vi "Create Index Map of Edges.vi"(8 "error in (no error)":errorcluster, 11 "2D Array binary in":refnum<class "2D Array binary.lvclass">) -> (0 "error out":errorcluster, 3 "2D Array binary out":refnum<class "2D Array binary.lvclass">)   [LabVIEW 2024, in "G2CPU Line Profile.lvlib"]
uses:
  G2CPU Line Profile.lvlib
  <vilib>/Natan Biesmans/G2CPU GPU and CPU HPC Toolkit/G2CPU Libraries/Arrays/2DArray/binary/2D Array binary.lvclass
  C:/Program Files/National Instruments/LabVIEW 2025/vi.lib/Natan Biesmans/G2CPU GPU and CPU HPC Toolkit/G2CPU Libraries/Arrays/Array/Array Prototype.lvclass
  C:/Program Files/National Instruments/LabVIEW 2025/vi.lib/Natan Biesmans/G2CPU GPU and CPU HPC Toolkit/G2CPU Libraries/Arrays/2DArray/2D Array Prototype.lvclass
  7be18b7c-d882-49a8-9bf3-9473975a2643.vi
  755dcc6d-d8b2-44ca-8967-bbed7c2483ca.vi
  b529d340-ea47-4164-86f1-e656114a860c.vi
  e5d4ff20-5dd6-4683-aa2a-8e7ba50b1f3d.vi
  d67c9315-a3db-4bd2-ba9f-b6b2c326ac84.vi
  a1422bdd-7d02-45b2-bd73-1aa3fc453463.vi
  be544eb2-5529-4343-82fc-932d6cc08acc.vi
  9e079d64-024a-4165-b95c-f022ae12d1bc.vi
  bbe568f6-b578-42fd-8d12-2a0471a10e1d.vi
  7be18b7c-d882-49a8-9bf3-9473975a2643.vi/e7247370-a01f-465a-ac0e-4dfefcb1bb87.vi
  7be18b7c-d882-49a8-9bf3-9473975a2643.vi/345e91f0-9a5e-4de4-af9c-133346717e4a.vi
  755dcc6d-d8b2-44ca-8967-bbed7c2483ca.vi/08cb2c43-1c8b-4a3a-83bc-b3e8cdef0e3a.vi
  755dcc6d-d8b2-44ca-8967-bbed7c2483ca.vi/f755307d-5806-43cd-9fa2-5ac75ab59def.vi
  755dcc6d-d8b2-44ca-8967-bbed7c2483ca.vi/37397dd5-2c89-4701-b050-64d2f1e61e81.vi
  b529d340-ea47-4164-86f1-e656114a860c.vi/e2b7cdad-9748-47a9-8803-19dad6ab3e2b.vi
  b529d340-ea47-4164-86f1-e656114a860c.vi/edeb7e37-ba5b-4522-b7cc-59d3333e22dd.vi
  e5d4ff20-5dd6-4683-aa2a-8e7ba50b1f3d.vi/f4654d05-beb0-4753-bab7-24376daae318.vi
  e5d4ff20-5dd6-4683-aa2a-8e7ba50b1f3d.vi/a2f9e1c9-c94e-4cd6-9432-cf54c3ac582a.vi
  d67c9315-a3db-4bd2-ba9f-b6b2c326ac84.vi/5fd79b99-6405-4116-b267-99be9ebfbdc8.vi
  d67c9315-a3db-4bd2-ba9f-b6b2c326ac84.vi/f56d75f8-a737-48e1-b5f1-0ddebb8102b6.vi
  d67c9315-a3db-4bd2-ba9f-b6b2c326ac84.vi/f51773da-75cb-4248-9bbd-2a32f0924584.vi
  d67c9315-a3db-4bd2-ba9f-b6b2c326ac84.vi/1de671e1-a703-4849-b735-ab080ea3bfc0.vi
  a1422bdd-7d02-45b2-bd73-1aa3fc453463.vi/f4654d05-beb0-4753-bab7-24376daae318.vi
  a1422bdd-7d02-45b2-bd73-1aa3fc453463.vi/a2f9e1c9-c94e-4cd6-9432-cf54c3ac582a.vi
  9e079d64-024a-4165-b95c-f022ae12d1bc.vi/e9bebd79-1c27-4fc1-b91f-30516104c7f0.vi
  bbe568f6-b578-42fd-8d12-2a0471a10e1d.vi/51c1d4c7-dece-4c02-9cce-b98611dadc4a.vi
  bbe568f6-b578-42fd-8d12-2a0471a10e1d.vi/3d9751b5-328d-444c-aff4-1d084998b389.vi
  b529d340-ea47-4164-86f1-e656114a860c.vi/e2b7cdad-9748-47a9-8803-19dad6ab3e2b.vi/6058dca8-195d-4566-b47b-6d6a1c5af61f.vi
  b529d340-ea47-4164-86f1-e656114a860c.vi/e2b7cdad-9748-47a9-8803-19dad6ab3e2b.vi/6058dca8-195d-4566-b47b-6d6a1c5af61f.vi/77c7badc-ed81-4514-99c1-20d37f4e5ecc.vi
  b529d340-ea47-4164-86f1-e656114a860c.vi/e2b7cdad-9748-47a9-8803-19dad6ab3e2b.vi/6058dca8-195d-4566-b47b-6d6a1c5af61f.vi/eb76fa01-6782-47b4-b34f-9eb474c9cc78.vi
  <vilib>/Natan Biesmans/G2CPU GPU and CPU HPC Toolkit/G2CPU Libraries/Arrays/2DArray/s64/2D Array s64.lvclass
  <vilib>/Natan Biesmans/G2CPU GPU and CPU HPC Toolkit/G2CPU Libraries/Arrays/2DArray/2D Array Prototype.lvclass
  <vilib>/Natan Biesmans/G2CPU GPU and CPU HPC Toolkit/G2CPU Libraries/Arrays/1DArray/binary/1D Array binary.lvclass
  <vilib>/Natan Biesmans/G2CPU GPU and CPU HPC Toolkit/G2CPU Libraries/Arrays/Array/G2CPU Get Array Pointer.vi
  <vilib>/Natan Biesmans/G2CPU GPU and CPU HPC Toolkit/ArrayFire Driver/VIs/cast.vi
  <vilib>/Natan Biesmans/G2CPU GPU and CPU HPC Toolkit/G2CPU Libraries/Arrays/Array/G2CPU Set Array Pointer.vi
  <vilib>/Natan Biesmans/G2CPU GPU and CPU HPC Toolkit/G2CPU Libraries/Arrays/Array/G2CPU Unlock Array.vi
  <vilib>/Natan Biesmans/G2CPU GPU and CPU HPC Toolkit/G2CPU Libraries/Arrays/Array/G2CPU Release Array.vi
  <vilib>/Natan Biesmans/G2CPU GPU and CPU HPC Toolkit/G2CPU Libraries/Arrays/Array/G2CPU Lock Array.vi
  <vilib>/Natan Biesmans/G2CPU GPU and CPU HPC Toolkit/ArrayFire Driver/VIs/diff1.vi
  <vilib>/Natan Biesmans/G2CPU GPU and CPU HPC Toolkit/ArrayFire Driver/VIs/Run as Multi Device.vi
  <vilib>/Natan Biesmans/G2CPU GPU and CPU HPC Toolkit/ArrayFire Driver/VIs/iszero.vi
  <vilib>/Natan Biesmans/G2CPU GPU and CPU HPC Toolkit/ArrayFire Driver/VIs/sub.vi
  <vilib>/Natan Biesmans/G2CPU GPU and CPU HPC Toolkit/ArrayFire Driver/VIs/release array.vi
  <vilib>/Natan Biesmans/G2CPU GPU and CPU HPC Toolkit/G2CPU Libraries/Manage Environment/Find AF DLL.vi
  <vilib>/Natan Biesmans/G2CPU GPU and CPU HPC Toolkit/ArrayFire Driver/subvi/Error Converter (ErrCode or Status).vi
  <vilib>/Natan Biesmans/G2CPU GPU and CPU HPC Toolkit/ArrayFire Driver/VIs/add.vi
  <vilib>/Natan Biesmans/G2CPU GPU and CPU HPC Toolkit/G2CPU Libraries/Arrays/SubVI/Lock Arrays.vi
  <vilib>/Natan Biesmans/G2CPU GPU and CPU HPC Toolkit/ArrayFire Driver/VIs/eq.vi
  <vilib>/Natan Biesmans/G2CPU GPU and CPU HPC Toolkit/ArrayFire Driver/VIs/not.vi
  <vilib>/Natan Biesmans/G2CPU GPU and CPU HPC Toolkit/ArrayFire Driver/VIs/any true.vi
  <vilib>/Natan Biesmans/G2CPU GPU and CPU HPC Toolkit/G2CPU Libraries/Arrays/SubVI/RemoveReducedDimensionForReorder.vi
  <vilib>/Natan Biesmans/G2CPU GPU and CPU HPC Toolkit/ArrayFire Driver/VIs/reorder.vi
  <vilib>/Natan Biesmans/G2CPU GPU and CPU HPC Toolkit/G2CPU Libraries/Arrays/Array/G2CPU Get Array Pointer Reference.vi
  <vilib>/Natan Biesmans/G2CPU GPU and CPU HPC Toolkit/G2CPU Libraries/Arrays/Array/G2CPU Set Array Pointer Reference.vi
  <vilib>/Natan Biesmans/G2CPU GPU and CPU HPC Toolkit/ArrayFire Driver/VIs/transpose.vi
  <vilib>/Natan Biesmans/G2CPU GPU and CPU HPC Toolkit/ArrayFire Driver/VIs/join.vi
  <vilib>/Natan Biesmans/G2CPU GPU and CPU HPC Toolkit/G2CPU Libraries/Arrays/Array/Array Prototype.lvclass
  <vilib>/Natan Biesmans/G2CPU GPU and CPU HPC Toolkit/G2CPU Libraries/Arrays/DataTypes/I64/s64.lvclass
  <vilib>/Natan Biesmans/G2CPU GPU and CPU HPC Toolkit/G2CPU Libraries/Arrays/DataTypes/Boolean/Boolean.lvclass
  <vilib>/Natan Biesmans/G2CPU GPU and CPU HPC Toolkit/G2CPU Libraries/Arrays/1DArray/1D Array Prototype.lvclass
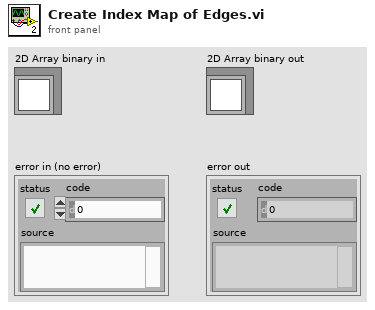
[diagram p1: front panel]
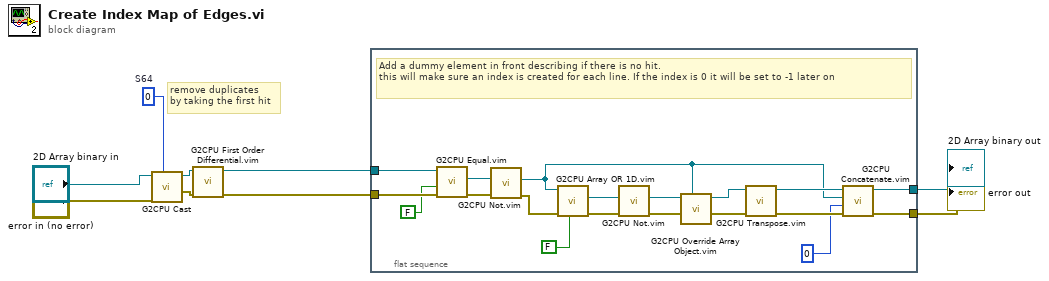
[diagram p0: block diagram]
diagram:
  w9 = i64 0  # S64
  # "remove duplicates\nby taking the first hit"
  n1 = call "G2CPU Cast"("Datatype Prototype"=w9, "error in (no error)"="error in (no error)", "Array In"="2D Array binary in") -> ("error out"=w2:errorcluster, "Array Out"=w3:refnum<class "2D Array s64.lvclass">)  [unwired: 7 in]
  n2 = call "G2CPU First Order Differential.vim"("error in (no error)"=w2, "Array in"=w3) -> ("error out"=w7:errorcluster, "Array Result"=w8:refnum<class "2D Array s64.lvclass">)  [unwired: 8 in]
  n3 = flat-sequence {
    tunnel: [w24] -> w5
    tunnel: [w19] -> w6
    tunnel: w7 -> [w14]
    tunnel: w8 -> [w13]
    frame #0 {
      # "Add a dummy element in front describing if there is no hit.\nthis will make sure an index is created for each line. If the index is 0 it will be set to -1 later on"
      n4 = call "G2CPU Equal.vim"("error in (no error)"=w14, "Array rhs"=FALSE ("Auto Release lhs (Enabled)"), "Array lhs"=w13) -> ("error out"=w12:errorcluster, "Array Result"=w11:refnum<class "2D Array binary.lvclass">)  [unwired: 7 in]
      n5 = call "G2CPU Not.vim"("error in (no error)"=w12, "Array in"=w11) -> ("error out"=w15:errorcluster, "Array Result"=w23:refnum<class "2D Array binary.lvclass">)  [unwired: 8 in]
      n6 = call "G2CPU Array OR 1D.vim"("Auto Release (Enabled)"=FALSE, "error in (no error)"=w15, "Array First"=w23) -> ("error out"=w16:errorcluster, "Array Result"=w18:refnum<class "1D Array binary.lvclass">)  [unwired: 7 in]
      n7 = call "G2CPU Not.vim"("error in (no error)"=w16, "Array in"=w18) -> ("error out"=w21:errorcluster, "Array Result"=w20:refnum<class "1D Array binary.lvclass">)  [unwired: 8 in]
      n8 = call "G2CPU Override Array Object.vim"("New Array Type"=w23, "error in (no error)"=w21, "To Override Array"=w20) -> ("error out"=w26:errorcluster, "Overriden Array (inplace)"=w25:refnum<class "2D Array binary.lvclass">)  [unwired: 7 in]
      n9 = call "G2CPU Transpose.vim"("error in (no error)"=w26, "Array In"=w25) -> ("error out"=w28:errorcluster, "Array out"=w27:refnum<class "2D Array binary.lvclass">)  [unwired: 8 in]
      n10 = call "G2CPU Concatenate.vim"("error in (no error)"=w28, "dim to join"=0, "Second Array In"=w23, "First Array In"=w27) -> ("error out"=w24:errorcluster, "Array out"=w19:refnum<class "2D Array binary.lvclass">)  [unwired: 6 in]
    }
  }
  "2D Array binary out" <- w6
  "error out" <- w5
